vi "encodeArrayHeader.vi"(3 "Number of Elements":u32) -> (1 "array header":u8[](array[numeric]) format="%.0x")   [LabVIEW 2015, in "MsgPack.lvlib"]
uses:
  MsgPack.lvlib
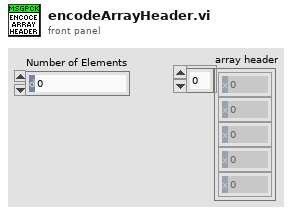
[diagram p1: front panel]
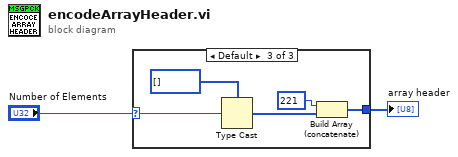
[diagram p0: block diagram]
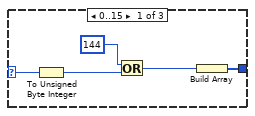
[diagram p2: hidden frame]
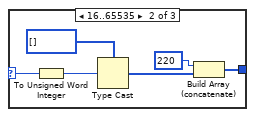
[diagram p3: hidden frame]
diagram:
  n1 = case shown="Default" "Number of Elements" {
    selector: "Number of Elements" -> [w5 w13 w14]
    tunnel: [w3 w8 w15] -> w2
    frame 0..15 {
      n2 = To Unsigned Byte Integer(number=w5) -> (unsigned 8bit integer=w7:u8)
      n3 = Or(x=u8 144, y=w7) -> (x .or. y?=w4:u8)
      n4 = Build Array(w4) -> (w3:u8[])
    }
    frame 16..65535 {
      n5 = To Unsigned Word Integer(number=w13) -> (unsigned 16bit integer=w11:u16)
      n6 = Type Cast(type=u8[] [], x=w11) -> (*(type *) &x=w9:u8[])
      n7 = Build Array (concatenate)(u8 220 ("x"), w9) -> (w8:u8[])
    }
    frame Default {
      n8 = Type Cast(type=u8[] [], x=w14) -> (*(type *) &x=w18:u8[])
      n9 = Build Array (concatenate)(u8 221 ("x"), w18) -> (w15:u8[])
    }
  }
  "array header" <- w2
